vi "move.vi"(8 "error in (no error)":errorcluster, 11 "MH100301DMC in":refnum<class "StageMH100301DMC.lvclass">) -> (0 "error out":errorcluster, 3 "MH100301DMC out":refnum<class "StageMH100301DMC.lvclass">)   [LabVIEW 2010, in "StageMH100301DMC.lvclass"]
uses:
  StageMH100301DMC.lvclass
  StageDL090409Scaffold/StageDL090409Scaffold/StageDL090409Scaffold.lvclass
  common/classes/ErrorController/ErrorController/class_data.vi
  common/classes/ErrorController/ErrorController/ErrorController.lvclass
  common/classes/SpaceVector/SpaceVector/SpaceVector.lvclass
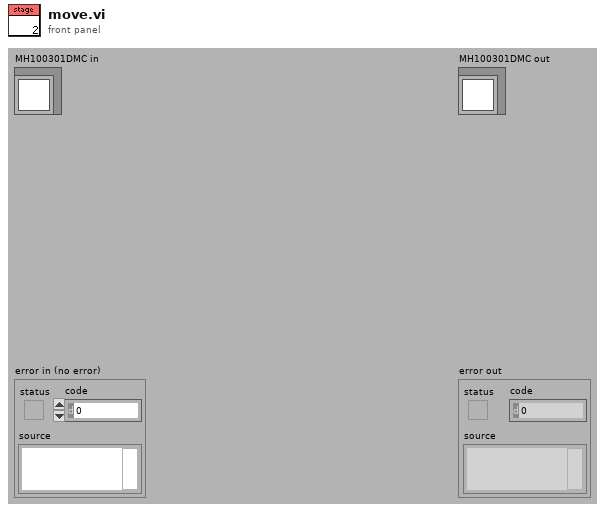
[diagram p1: front panel]
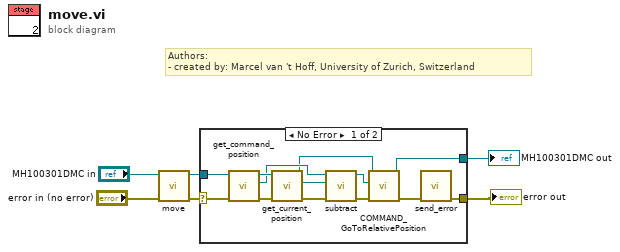
[diagram p0: block diagram]
diagram:
  # "Authors: \n- created by: Marcel van 't Hoff, University of Zurich, Switzerland"
  n1 = call-parent "move.vi"("error in (no error)"="error in (no error)", "DL090409StageScaffold in"="MH100301DMC in") -> ("error out"=w2:errorcluster, "DL090409StageScaffold out"=w1:refnum<class "StageMH100301DMC.lvclass">)  [unwired: 8 out]
  n2 = case shown="No Error" w2 {
    selector: w2 -> [w13 w21]
    tunnel: [w16 w21] -> w6
    tunnel: [w18 w20] -> w5
    tunnel: w1 -> [w19 w20]
    frame No Error {
      n3 = call-dynamic "get_command_position.vi"("error in (no error)"=w13, "DL090409StageScaffold.lvclass in"=w19) -> ("error out"=w15:errorcluster, "SpaceVector.lvclass"=w12:refnum<class "SpaceVector.lvclass">, "DL090409StageScaffold.lvclass out"=w14:refnum<class "StageMH100301DMC.lvclass">)  [unwired: 7 out]
      n4 = call-dynamic "get_current_position.vi"("error in (no error)"=w15, "DL090409StageScaffold.lvclass in"=w14) -> ("error out"=w10:errorcluster, "current position"=w11:refnum<class "SpaceVector.lvclass">, "DL090409StageScaffold.lvclass out"=w7:refnum<class "StageMH100301DMC.lvclass">)  [unwired: 7 in]
      n5 = call "subtract.vi"("error in (no error)"=w10, "subtrahend"=w11, "SpaceVector in"=w12) -> ("error out"=w9:errorcluster, "SpaceVector out"=w8:refnum<class "SpaceVector.lvclass">)  [unwired: 7 in]
      n6 = call-dynamic "COMMAND_GoToRelativePosition.vi"("error in (no error)"=w9, "target  position"=w8, "MH100301DMC in"=w7) -> ("error out"=w17:errorcluster, "MH100301DMC out"=w18:refnum<class "StageMH100301DMC.lvclass">)  [unwired: 7 in]
      n7 = call "send_error.vi"("error in (no error)"=w17) -> ("error out"=w16:errorcluster)  [unwired: 10 in]
    }
    frame Error {
    }
  }
  "error out" <- w6
  "MH100301DMC out" <- w5
